vi "Sistema de Movimiento para Focalizar Punta.vi"(0 "Micras en X":dbl, 1 "Micras en Y":dbl, 2 "Micras en Z":dbl, 3 "Activar movimiento en X":bool, 4 "Activar movimiento en Y":bool, 5 "Activar movimiento en Z":bool, 6 "Caso de Entrada":i32, 7 "error in":errorcluster, 8 "VISA Micro XY":refnum<visa-resource-name>, 9 "VISA Micro Z":refnum<visa-resource-name>) -> (14 "Caso de salida":i32, 16 "VISA resource name out":refnum<visa-resource-name>, 17 "VISA resource name out 2":refnum<visa-resource-name>, 18 "error out Z":errorcluster, 19 "error out XY":errorcluster)   [LabVIEW 2018]
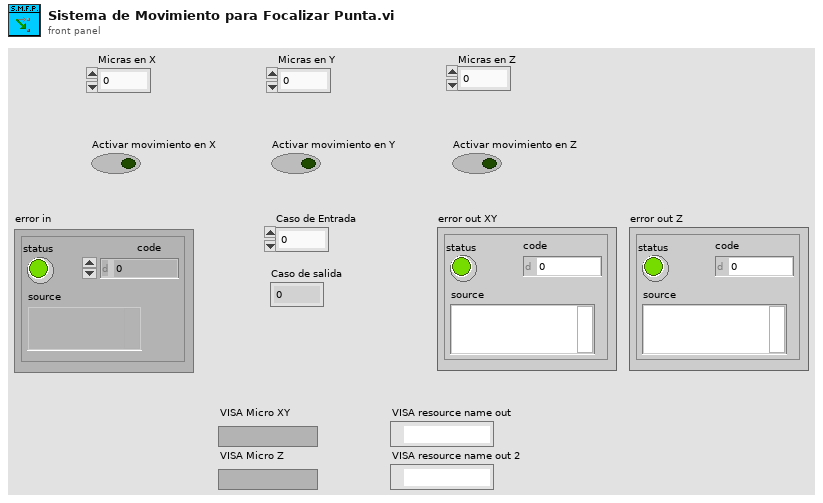
[diagram p1: front panel]
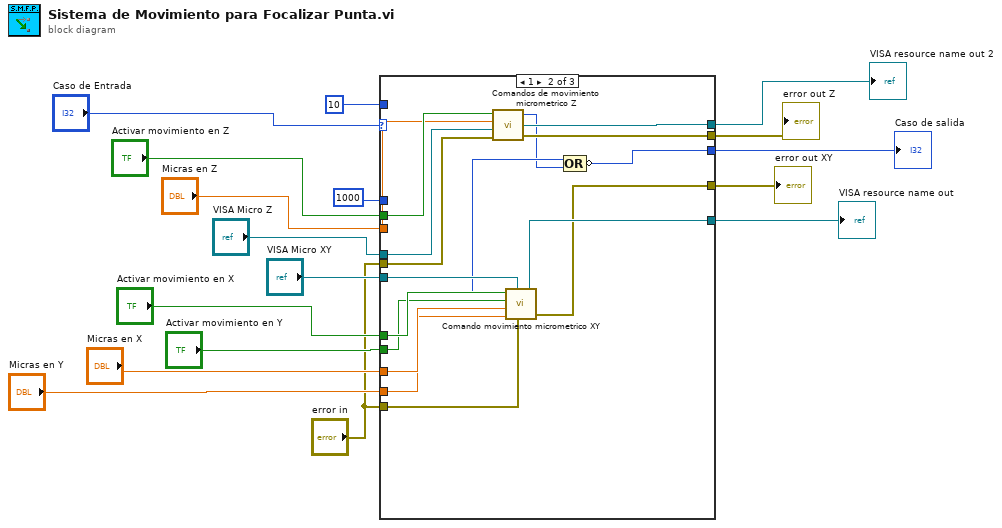
[diagram p0: block diagram]
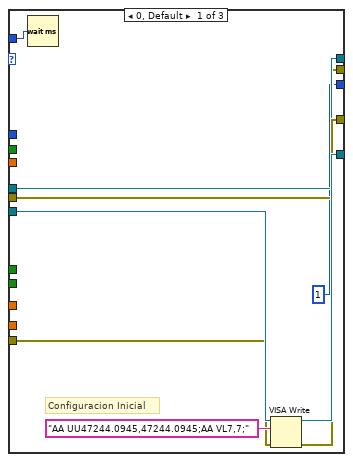
[diagram p2: hidden frame]
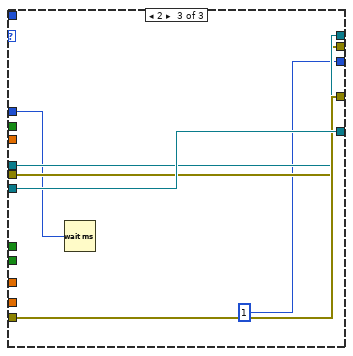
[diagram p3: hidden frame]
diagram:
  n1 = case shown="1" "Caso de Entrada" {
    tunnel: "VISA Micro XY" -> [w25 w37 w49]
    tunnel: "error in" -> [w24 w36 w48]
    tunnel: u32 10 -> [w23 _ _]
    tunnel: [w22 w35 w49] -> w15
    tunnel: [w21 w34 w48] -> w3
    tunnel: [w20 w41 w47] -> w14
    tunnel: "VISA Micro Z" -> [w20 w43 w47]
    tunnel: [w19 w40 w46] -> w2
    tunnel: "error in" -> [w19 w42 w46]
    tunnel: "Activar movimiento en Z" -> [_ w39 _]
    tunnel: "Micras en Z" -> [_ w38 _]
    tunnel: [1 w27 1] -> w12
    tunnel: "Activar movimiento en X" -> [_ w33 _]
    tunnel: "Activar movimiento en Y" -> [_ w32 _]
    tunnel: "Micras en X" -> [_ w31 _]
    tunnel: "Micras en Y" -> [_ w30 _]
    tunnel: u32 1000 -> [_ _ w44]
    frame 0, Default {
      # "Configuracion Inicial"
      n2 = Wait (ms)(milliseconds to wait=w23) -> ()  [unwired: 1 out]
      n3 = VISA Write(VISA resource name=w25, write buffer="AA UU47244.0945,47244.0945;AA VL7,7;", error in (no error)=w24) -> (VISA resource name out=w22:refnum<visa-resource-name>, error out=w21:errorcluster)  [unwired: 1 out]
    }
    frame 1 {
      n4 = call "Comandos de movimiento micrometrico Z.vi"("error in"=w42, "VISA in"=w43, "Micras en Z"=w38, "Activar Movimiento en Z"=w39) -> ("error out"=w40:errorcluster, "VISA out"=w41:refnum<visa-resource-name>, "Siguiente caso"=w28:i32)
      n5 = call "Comando movimiento micrometrico XY.vi"("Activar movimiento en X"=w33, "VISA resource name"=w37, "Activar movimiento en Y"=w32, "Micras en X"=w31, "error in"=w36, "Micras en Y"=w30) -> ("Caso"=w29:i32, "VISA resource name out"=w35:refnum<visa-resource-name>, "error out"=w34:errorcluster)
      n6 = Compound Arithmetic op=OR(w29, w28) -> (invert w27:i32)
    }
    frame 2 {
      n7 = Wait (ms)(milliseconds to wait=w44) -> ()  [unwired: 1 out]
    }
  }
  "error out XY" <- w3
  "Caso de salida" <- w12
  "VISA resource name out" <- w15
  "VISA resource name out 2" <- w14
  "error out Z" <- w2
